vi "testSendTelToClientAndCmdFromClient.vi"(8 "error in (no error)":errorcluster) -> (0 "error out":errorcluster)   [LabVIEW 2018]
doc: "This VI sends commands from TCP client and receives the Ack from TCP server. Besides, TCP server sends telemetry to TCP client."
uses:
  <vilib>/addons/_JKI Toolkits/Caraya/classes/Assert/Assert Equal Value_Variant.vi
  src/TcpServer/TcpServer.lvclass
  <vilib>/addons/_JKI Toolkits/Caraya/classes/Test/Test.lvclass
  <vilib>/addons/_JKI Toolkits/Caraya/classes/Assert/Assert.lvclass
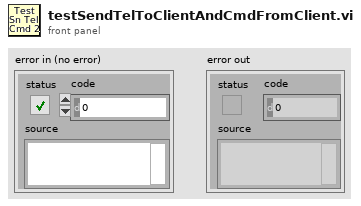
[diagram p1: front panel]
types:
  T1 = cluster{"CmdRead":refnum<user-event>, "EvtRead":refnum<user-event>, "GenRead":refnum<user-event>}
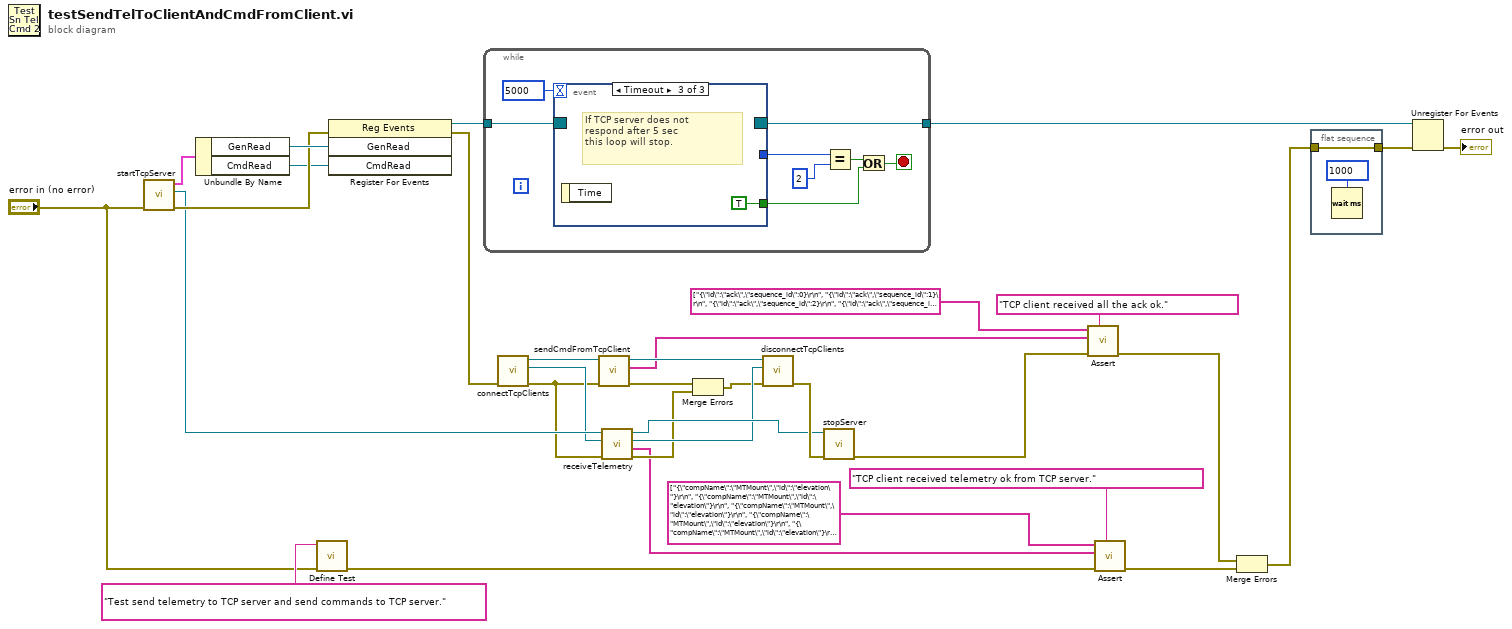
[diagram p0: block diagram]
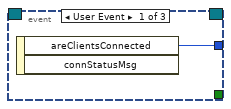
[diagram p2: hidden frame]
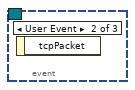
[diagram p3: hidden frame]
diagram:
  n1 = call "startTcpServer.vi"("error in (no error)"="error in (no error)") -> ("error out"=w26:errorcluster, "TcpServer out"=w11:refnum<class "TcpServer.lvclass">, "UserEvents"=w28:T1)  [unwired: 8 in]
  n2 = Unbundle By Name(w28) -> ("GenRead"=w27:refnum<user-event>, "CmdRead"=w17:refnum<user-event>)
  n3 = call <vilib>:"Define Test.vi"("error in (no error)"="error in (no error)", "Label (VI Title)"="Test send telemetry to TCP server and send commands to TCP server.") -> ("error out"=w24:errorcluster)  [unwired: 9 in]
  n4 = register-events(error in=w26, w27, w17) -> (reference out=w33:refnum<event-registration>, error out=w1:errorcluster)  [unwired: 1 in]
  n5 = while {
    tunnel: w33 -> [w41]
    tunnel: [w40] -> w32
    stop <- w37 stop-if-true
    n6 = event shown="[2] Timeout" {
      selector: w41 -> [_ _ _]
      dyn-events: [_ _ _] -> w40
      timeout: 5000 -> [_ _ _]
      tunnel: [w42 _ _] -> w39
      tunnel: [_ _ TRUE] -> w34
      event User Event {
        n7 = event-data() -> ("areClientsConnected"=w42:enum16{"unchanged", "connected", "unconnected"})  [unwired: 1 in, 1 out]
      }
      event User Event {
        n8 = event-data() -> ()  [unwired: 1 in, 1 out]
      }
      event Timeout {
        # "If TCP server does not\nrespond after 5 sec\nthis loop will stop."
        n9 = event-data() -> ()  [unwired: 1 in, 1 out]
      }
    }
    n10 = Equal?(x=w39, y=2) -> (x = y?=w35:bool)
    n11 = Or(x=w35, y=w34) -> (x .or. y?=w37:bool)
  }
  n12 = call "connectTcpClients.vi"("error in (no error)"=w1) -> ("error out"=w2:errorcluster, "tel connection ID out"=w9:refnum<k5>, "cmd connection ID out"=w20:refnum<k5>)  [unwired: 8 in]
  n13 = call "sendCmdFromTcpClient.vi"("error in (no error)"=w2, "connection ID in"=w20) -> ("error out"=w15:errorcluster, "ack received"=w12:string[], "connection ID out"=w16:refnum<k5>)  [unwired: 7 in]
  n14 = call "receiveTelemetry.vi"("error in (no error)"=w2, "tel connection in"=w9, "TcpServer out"=w11) -> ("error out"=w7:errorcluster, "telemetry received"=w6:string[], "tel connection out"=w8:refnum<k5>, "tcpServer out"=w10:refnum<class "TcpServer.lvclass">)  [unwired: 5 in]
  n15 = Merge Errors(w15, w7) -> (w4:errorcluster)
  n16 = call "disconnectTcpClients.vi"("error in (no error)"=w4, "tel connection ID in"=w8, "cmd connection ID in"=w16) -> ("error out"=w14:errorcluster)  [unwired: 8 in]
  n17 = call "stopServer.vi"("error in (no error)"=w14, "tcpServer in"=w10) -> ("error out"=w13:errorcluster)  [unwired: 8 in, 1 out]
  n18 = call-poly <vilib>:"Assert.vi"("Label"="TCP client received all the ack ok.", "error in (no error)"=w13, "Y"=w12, "X"=string[] ["{\"id\":\"ack\",\"sequence_id\":0}\r\n", "{\"id\":\"ack\",\"sequence_id\":1}\r\n", "{\"id\":\"ack\",\"sequence_id\":2}\r\n", "{\"id\":\"ack\",\"sequence_id\":6}\r\n", "{\"id\":\"noack\",\"sequence_id\":3}\r\n", "{\"id\":\"noack\",\"sequence_id\":4}\r\n", "{\"id\":\"noack\",\"sequence_id\":5}\r\n", "{\"id\":\"ack\",\"sequence_id\":7}\r\n", "{\"id\":\"ack\",\"sequence_id\":8}\r\n", "{\"id\":\"ack\",\"sequence_id\":9}\r\n"] ("ack received 2")) -> ("error out"=w18:errorcluster)  [unwired: 7 in]
  n19 = call-poly <vilib>:"Assert.vi"("Label"="TCP client received telemetry ok from TCP server.", "error in (no error)"=w24, "Y"=w6, "X"=string[] ["{\"compName\":\"MTMount\",\"id\":\"elevation\"}\r\n", "{\"compName\":\"MTMount\",\"id\":\"elevation\"}\r\n", "{\"compName\":\"MTMount\",\"id\":\"elevation\"}\r\n", "{\"compName\":\"MTMount\",\"id\":\"elevation\"}\r\n", "{\"compName\":\"MTMount\",\"id\":\"elevation\"}\r\n", "{\"compName\":\"MTMount\",\"id\":\"elevation\"}\r\n", "{\"compName\":\"MTMount\",\"id\":\"elevation\"}\r\n", "{\"compName\":\"MTMount\",\"id\":\"elevation\"}\r\n", "{\"compName\":\"MTMount\",\"id\":\"elevation\"}\r\n", "{\"compName\":\"MTMount\",\"id\":\"elevation\"}\r\n", "{\"compName\":\"MTMount\",\"id\":\"elevation\"}\r\n", "{\"compName\":\"MTMount\",\"id\":\"elevation\"}\r\n", "{\"compName\":\"MTMount\",\"id\":\"elevation\"}\r\n", "{\"compName\":\"MTMount\",\"id\":\"elevation\"}\r\n", "{\"compName\":\"MTMount\",\"id\":\"elevation\"}\r\n", "{\"compName\":\"MTMount\",\"id\":\"elevation\"}\r\n", "{\"compName\":\"MTMount\",\"id\":\"elevation\"}\r\n", "{\"compName\":\"MTMount\",\"id\":\"elevation\"}\r\n", "{\"compName\":\"MTMount\",\"id\":\"elevation\"}\r\n", "{\"compName\":\"MTMount\",\"id\":\"elevation\"}\r\n", "{\"compName\":\"MTMount\",\"id\":\"elevation\"}\r\n", "{\"compName\":\"MTMount\",\"id\":\"elevation\"}\r\n", "{\"compName\":\"MTMount\",\"id\":\"elevation\"}\r\n", "{\"compName\":\"MTMount\",\"id\":\"elevation\"}\r\n", "{\"compName\":\"MTMount\",\"id\":\"elevation\"}\r\n", "{\"compName\":\"MTMount\",\"id\":\"elevation\"}\r\n", "{\"compName\":\"MTMount\",\"id\":\"elevation\"}\r\n", "{\"compName\":\"MTMount\",\"id\":\"elevation\"}\r\n", "{\"compName\":\"MTMount\",\"id\":\"elevation\"}\r\n", "{\"compName\":\"MTMount\",\"id\":\"elevation\"}\r\n", "{\"compName\":\"MTMount\",\"id\":\"elevation\"}\r\n", "{\"compName\":\"MTMount\",\"id\":\"elevation\"}\r\n", "{\"compName\":\"MTMount\",\"id\":\"elevation\"}\r\n", "{\"compName\":\"MTMount\",\"id\":\"elevation\"}\r\n", "{\"compName\":\"MTMount\",\"id\":\"elevation\"}\r\n", "{\"compName\":\"MTMount\",\"id\":\"elevation\"}\r\n", "{\"compName\":\"MTMount\",\"id\":\"elevation\"}\r\n", "{\"compName\":\"MTMount\",\"id\":\"elevation\"}\r\n", "{\"compName\":\"MTMount\",\"id\":\"elevation\"}\r\n", "{\"compName\":\"MTMount\",\"id\":\"elevation\"}\r\n", "{\"compName\":\"MTMount\",\"id\":\"elevation\"}\r\n", "{\"compName\":\"MTMount\",\"id\":\"elevation\"}\r\n", "{\"compName\":\"MTMount\",\"id\":\"elevation\"}\r\n", "{\"compName\":\"MTMount\",\"id\":\"elevation\"}\r\n", "{\"compName\":\"MTMount\",\"id\":\"elevation\"}\r\n", "{\"compName\":\"MTMount\",\"id\":\"elevation\"}\r\n", "{\"compName\":\"MTMount\",\"id\":\"elevation\"}\r\n", "{\"compName\":\"MTMount\",\"id\":\"elevation\"}\r\n", "{\"compName\":\"MTMount\",\"id\":\"elevation\"}\r\n", "{\"compName\":\"MTMount\",\"id\":\"elevation\"}\r\n"] ("Array 2")) -> ("error out"=w21:errorcluster)  [unwired: 7 in]
  n20 = Merge Errors(w18, w21) -> (w22:errorcluster)
  n21 = flat-sequence {
    tunnel: w22 -> [w44]
    tunnel: [w44] -> w30
    frame #0 {
      n22 = Wait (ms)(milliseconds to wait=u32 1000) -> ()  [unwired: 1 out]
    }
  }
  n23 = Unregister For Events(event registration refnum=w32, error in=w30) -> (error out=→"error out":errorcluster)
